vi "fxp_PID.vi"(0 "process variable":fxp<+/-,16,9>, 1 "reset?":bool, 7 "setpoint":fxp<+/-,16,9>, 12 "PID gains":T2={"proportional gain (Kc)"=3.0, "integral gain (Kc*Ts/Ti)"=0.0, "derivative gain (Kc*Td/Ts)"=19.796875}, 13 "output range":T1={"output high"=180.0, "output low"=-180.0}) -> (4 "output":fxp<+/-,16,9>)   [LabVIEW 2016]
doc: "On an FPGA target, implements an integer PID algorithm for PID applications with high-speed control and/or high channel count that require an efficient algorithm. You can use this Express VI with single-channel or multi-channel configurations. The PID algorithm features control action range and uses the integrator anti-windup calculation to limit the effect of the integral action during transients. The PID algorithm also features bumpless controller output for PID gain changes.\n--------------------\n\nThis Express VI is configured as follows:\n\nNumber of channels = 1\nProportional gain (Kc) = 3\nIntegral time (Ti) = 0 min\nDerivative time (Td) = 0.00109993 min\nSampling time (Ts) = 0.01 s\nProportional gain (normalized) (Kc) = 3\nIntegral gain (normalized) ([Kc*Ts]/[Ti*60]) = 0\nDerivative gain (normalized) ([Kc*Td*60]/[Ts]) = 19.7969\nOutput range high = 180\nOutput range low = -180\nInitial setpoint = 0"
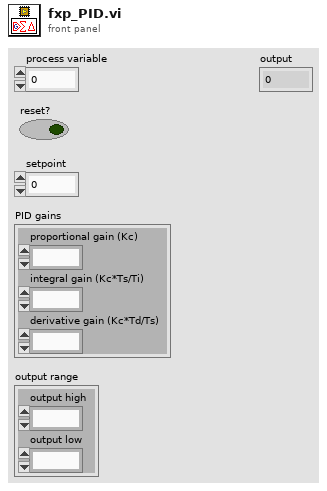
[diagram p1: front panel]
types:
  T1 = cluster{"output high":fxp<+/-,16,9>, "output low":fxp<+/-,16,9>}
  T2 = cluster{"proportional gain (Kc)":fxp<+/-,16,8>, "integral gain (Kc*Ts/Ti)":fxp<+/-,16,8>, "derivative gain (Kc*Td/Ts)":fxp<+/-,16,8>}
  T3 = cluster{"proportional gain (Kc)":i16, "integral gain (Kc*Ts/Ti)":i16, "derivative gain (Kc*Td/Ts)":i16}
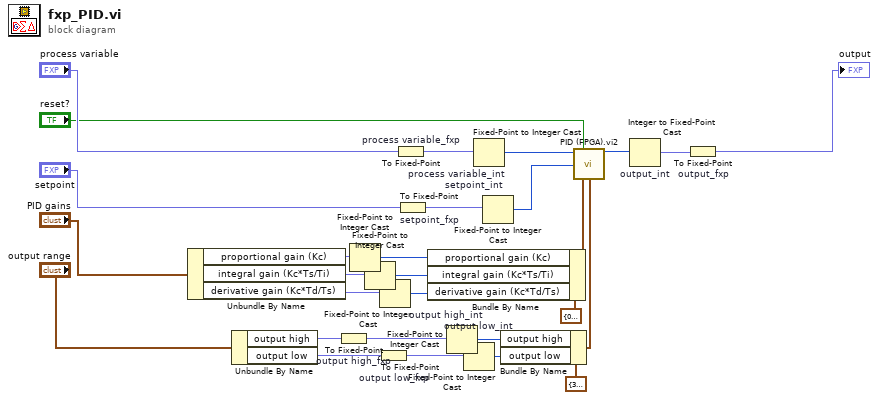
[diagram p0: block diagram]
diagram:
  n1 = Unbundle By Name("PID gains") -> ("proportional gain (Kc)"=w14:fxp<+/-,16,8>, "integral gain (Kc*Ts/Ti)"=w15:fxp<+/-,16,8>, "derivative gain (Kc*Td/Ts)"=w16:fxp<+/-,16,8>)
  n2 = Unbundle By Name("output range") -> ("output high"=w2:fxp<+/-,16,9>, "output low"=w1:fxp<+/-,16,9>)
  n3 = To Fixed-Point "output high_fxp"(number=w2) -> (fixed-point=w17:fxp<+/-,16,9>)  [unwired: 1 in]
  n4 = Fixed-Point to Integer Cast(1:w14) -> (0:w12:i16)
  n5 = Fixed-Point to Integer Cast(1:w15) -> (0:w13:i16)
  n6 = To Fixed-Point "output low_fxp"(number=w1) -> (fixed-point=w20:fxp<+/-,16,9>)  [unwired: 1 in]
  n7 = Fixed-Point to Integer Cast(1:w16) -> (0:w11:i16)
  n8 = To Fixed-Point "process variable_fxp"(number="process variable") -> (fixed-point=w8:fxp<+/-,16,9>)  [unwired: 1 in]
  n9 = To Fixed-Point "setpoint_fxp"(number="setpoint") -> (fixed-point=w9:fxp<+/-,16,9>)  [unwired: 1 in]
  n10 = Bundle By Name(cluster=T3 {"proportional gain (Kc)"=0, "integral gain (Kc*Ts/Ti)"=0, "derivative gain (Kc*Td/Ts)"=0} ("PID gains"), "proportional gain (Kc)"=w12, "integral gain (Kc*Ts/Ti)"=w13, "derivative gain (Kc*Td/Ts)"=w11) -> (w5:T3)
  n11 = Fixed-Point to Integer Cast "output high_int"(1:w17) -> (0:w18:i16)
  n12 = Fixed-Point to Integer Cast "output low_int"(1:w20) -> (0:w19:i16)
  n13 = Fixed-Point to Integer Cast "process variable_int"(1:w8) -> (0:w7:i16)
  n14 = Fixed-Point to Integer Cast "setpoint_int"(1:w9) -> (0:w10:i16)
  n15 = Bundle By Name(cluster=cluster{"output high":i16, "output low":i16} {"output high"=32767, "output low"=-32768} ("output range"), "output high"=w18, "output low"=w19) -> (w6:cluster{"output high":i16, "output low":i16})
  n16 = call "PID (FPGA).vi2"("process variable"=w7, "reset?"="reset?", "setpoint"=w10, "PID gains"=w5, "output range"=w6) -> ("output"=w21:i16)  [unwired: 10 in]
  n17 = Integer to Fixed-Point Cast "output_int"(integer=w21) -> (fixed-point=w22:fxp<+/-,16,9>)  [unwired: 1 in]
  n18 = To Fixed-Point "output_fxp"(number=w22) -> (fixed-point=→"output":fxp<+/-,16,9>)  [unwired: 1 in]
